vi "Servo MSMT Set Servo Type in Measurement Name.vi"(8 "error in (no error)":errorcluster, 11 "Input Power Measurement in":refnum<class "Input Power Measurement.lvclass">) -> (0 "error out":errorcluster, 3 "Input Power Measurement out":refnum<class "Input Power Measurement.lvclass">)   [LabVIEW 2018, in "Input Power Measurement.lvlib" / "Input Power Measurement.lvclass"]
uses:
  Input Power Measurement.lvclass
  C:/Sequence Automation/Plugins/Measurement Interface.lvlibp/Measurement Interface.lvclass
  Plugins/Measurement Interface.lvlibp/Private Methods/Measurement Name/Read Measurement Name.vi
  Plugins/Measurement Interface.lvlibp/Private Methods/Measurement Name/Write Measurement Name.vi
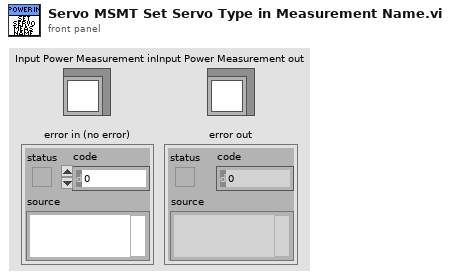
[diagram p1: front panel]
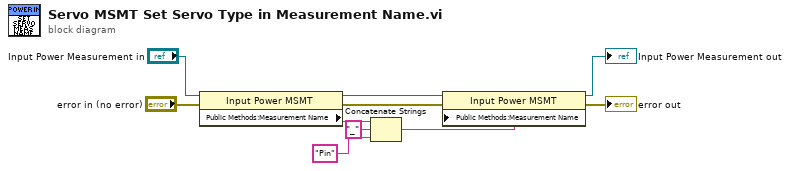
[diagram p0: block diagram]
diagram:
  n1 = property class="Input Power MSMT"(reference="Input Power Measurement in", error in="error in (no error)") -> (reference out=w5:refnum<class "Input Power Measurement.lvclass">, error out=w9:errorcluster, "Public Methods:Measurement Name"=w7:string)
  n2 = Concatenate Strings(w7, "_" ("string"), "Pin" ("string")) -> (w3:string)
  n3 = property class="Input Power MSMT"(reference=w5, error in=w9, "Public Methods:Measurement Name"=w3) -> (reference out=→"Input Power Measurement out":refnum<class "Input Power Measurement.lvclass">, error out=→"error out":errorcluster)
